vi "Begin.vi"(8 "error in":errorcluster) -> (0 "error out":errorcluster)   [LabVIEW 2017]
doc: "Called before other user functions, this VI is expected to open initial I/O refnums, load in file data, and do all program initialization. Notice that the <B>error out</B> terminal is simply used for data flow. Wiring it to other structures or subVIs ensures that this VI runs first."
uses:
  <vilib>/Rock Robotics/WPI/DriverStation/WPI_DriverStationRobotMode2.ctl
  <vilib>/Rock Robotics/WPI/Joystick/WPI_JoystickDeviceEnum.ctl
  <vilib>/Rock Robotics/WPI/ThirdParty/Phoenix-LabVIEW/Motor Controller/Controls/CTRE_Phoenix_MotorControl_ControlMode.ctl
  <vilib>/Rock Robotics/WPI/ThirdParty/Phoenix-LabVIEW/CANifier/CTRE_CANifier_StatusFrame.ctl
  <vilib>/Rock Robotics/WPI/ThirdParty/Phoenix-LabVIEW/Motor Controller/Controls/CTRE_Phoenix_MotorControl_FeedbackDevice.ctl
  Robot Global Data.vi
  <vilib>/Rock Robotics/WPI/ThirdParty/Phoenix-LabVIEW/Pigeon IMU/CTRE_PigeonIMU_Open_CAN.vi
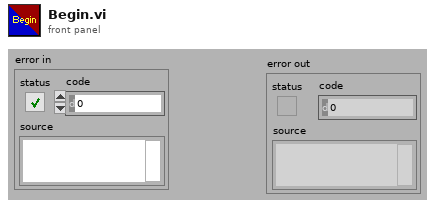
[diagram p1: front panel]
types:
  T1 = typedef "CTRE_Phoenix_MotorControl_FeedbackDevice.ctl" = i8
  T2 = typedef "CTRE_CANifier_StatusFrame.ctl" = u32
  T3 = typedef "CTRE_Phoenix_MotorControl_ControlMode.ctl" = u16
  T4 = typedef "WPI_JoystickDeviceEnum.ctl" = enum16{"USB 0", "USB 1", "USB 2", "USB 3", "USB 4", "USB 5"}
  T5 = typedef "WPI_DriverStationRobotMode2.ctl" = enum16{"Autonomous Disabled", "Autonomous Enabled", "Teleop Disabled", "Teleop Enabled", "Disconnected", "Finish", "Test Disabled", "Test Enabled", "Emergency Stopped"}
  T6 = typedef "WPI_JoystickDevRef.ctl" = cluster{"Device":T4}
  T7 = typedef "CTRE_PigeonIMU_DeviceRef.ctl" = cluster{"DeviceStatus":errorcluster, "Device Number":u8, "Type":T8, "Device ID":u32, "Handle":u64, "UsageFrame":u32, "Library Path":path}
  T8 = typedef "CTRE_PigeonIMU_ConnectionType.ctl" = u32
  T9 = typedef "WPI_MotorControlDeviceRef.ctl" = cluster{"DeviceStatus":errorcluster, "Type":T10, "PWM":cluster{"PWM Channel":T11, "DeadBand":T12}, "CAN":cluster{"Device Number":u8, "SetOutput VI Ref":variant, "GetOutput VI Ref":variant, "Enable VI Ref":variant, "Disable VI Ref":variant, "Data":variant}, "Invert":bool, "DIO PWM":cluster{"PWM \"Enable\" Channel":T11, "DIOChannel":T13, "PWM Rate":dbl}}
  T10 = typedef "WPI_MotorControlType.ctl" = enum16{"PWM", "CAN", "DIO PWM"}
  T11 = typedef "FPGA_DIOPWMChannel.ctl" = enum8{"PWM 0", "PWM 1", "PWM 2", "PWM 3", "PWM 4", "PWM 5", "PWM 6", "PWM 7", "PWM 8", "PWM 9", "PWM MXP 0", "PWM MXP 1", "PWM MXP 2", "PWM MXP 3", "PWM MXP 4", "PWM MXP 5", "PWM MXP 6", "PWM MXP 7", "PWM MXP 8", "PWM MXP 9", "Invalid"}
  T12 = typedef "WPI_PWMDeadband.ctl" = cluster{"Name":string, "maxPositivePwm":i32, "minPositivePwm":i32, "centerPwm":i32, "maxNegativePwm":i32, "minNegativePwm":i32, "angularRange":u16}
  T13 = typedef "FPGA_DIOChannel.ctl" = enum8{"DIO 0", "DIO 1", "DIO 2", "DIO 3", "DIO 4", "DIO 5", "DIO 6", "DIO 7", "DIO 8", "DIO 9", "DIO MXP 0", "DIO MXP 1", "DIO MXP 2", "DIO MXP 3", "DIO MXP 4", "DIO MXP 5", "DIO MXP 6", "DIO MXP 7", "DIO MXP 8", "DIO MXP 9", "DIO MXP 10", "DIO MXP 11", "DIO MXP 12", "DIO MXP 13", "DIO MXP 14", "DIO MXP 15", "SPI Port CS1", "SPI Port CS2", "SPI Port CS3", "SPI Port MISO", "SPI Port MOSI", "Invalid"}
  T14 = typedef "CTRE_CANifier_DeviceRef.ctl" = cluster{"DeviceStatus":errorcluster, "Device Number":u8, "Handle":u64, "UsageFrame":u32, "Library Path":path}
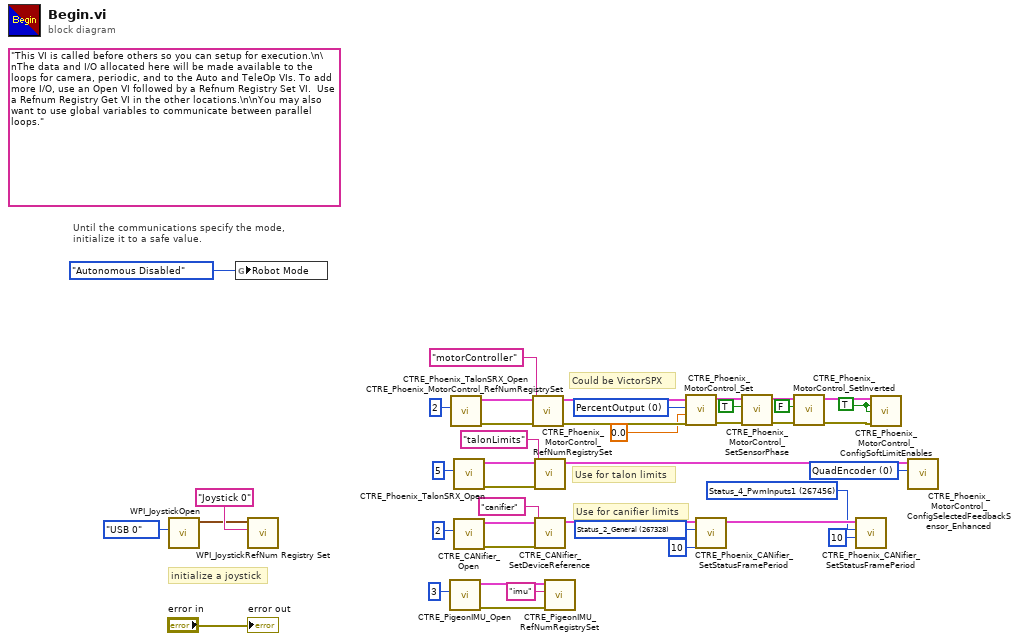
[diagram p0: block diagram]
diagram:
  w4 = T1 0 items=["None"=-1, "QuadEncoder"=0, "Analog"=2, "Tachometer"=4, "Pulse Width Encoded Position"=8, "Sensor Sum (S0 + S1)"=9, "Sensor Difference (D0 - D1)"=10, "Remote Source 0"=11, "Remote Source 1"=12, "Software Emulated"=15] ("Feedback Device")
  w1 = TRUE ("Override Soft Limit Enable?")
  w7 = T2 267456 items=["Status_1_General"=267264, "Status_2_General"=267328, "Status_3_PwmInputs0"=267392, "Status_4_PwmInputs1"=267456, "Status_5_PwmInputs2"=267520, "Status_6_PwmInputs3"=267584, "Status_8_Misc"=267712] ("CANifier Status Frame")
  w10 = T2 267328 items=["Status_1_General"=267264, "Status_2_General"=267328, "Status_3_PwmInputs0"=267392, "Status_4_PwmInputs1"=267456, "Status_5_PwmInputs2"=267520, "Status_6_PwmInputs3"=267584, "Status_8_Misc"=267712] ("CANifier Status Frame")
  w23 = T3 0 items=["PercentOutput"=0, "Position"=1, "Velocity"=2, "Current"=3, "Follower"=5, "MotionProfile"=6, "MotionMagic"=7, "MotionMagicArc"=8, "MotionProfileArc"=10, "Disabled"=15] ("Control Mode")
  (unwired) "This VI is called before others so you can setup for execution.\n\nThe data and I/O allocated here will be made available to the loops for camera, periodic, and to the Auto and TeleOp VIs. To add more I/O, use an Open VI followed by a Refnum Registry Set VI.  Use a Refnum Registry Get VI in the other locations.\n\nYou may also want to use global variables to communicate between parallel loops."
  # "Use for canifier limits"
  # "Use for talon limits"
  # "Could be VictorSPX"
  # "initialize a joystick"
  # "Until the communications specify the mode,\ninitialize it to a safe value."
  n1 = call <vilib>:"WPI_JoystickOpen.vi"("JoystickDevice"=WPI_JoystickDeviceEnum."USB 0") -> ("JoystickDevRef"=w40:T6)  [unwired: 10 in]
  n2 = global write "Robot Global Data.vi" "Robot Mode"(WPI_DriverStationRobotMode2."Autonomous Disabled" ("Robot Mode")) -> ()
  n3 = call <vilib>:"WPI_JoystickRefNum Registry Set.vi"("refnum name"="Joystick 0", "JoystickDevRef"=w40) -> ()  [unwired: 8 in, 2 out]
  n4 = call-poly <vilib>:"CTRE_PigeonIMU_Open.vi"("Device Number"=u8 3) -> ("error out"=w20:errorcluster, "PigeonIMUDevRef"=w19:T7)  [unwired: 9 in]
  n5 = call <vilib>:"CTRE_Phoenix_TalonSRX_Open.vi"("Device Number"=u8 2) -> ("error out"=w36:errorcluster, "CAN Talon SRX Ref"=w35:T9)  [unwired: 9 in]
  n6 = call <vilib>:"CTRE_Phoenix_TalonSRX_Open.vi"("Device Number"=u8 5) -> ("error out"=w32:errorcluster, "CAN Talon SRX Ref"=w31:T9)  [unwired: 9 in]
  n7 = call <vilib>:"CTRE_CANifier_Open.vi"("Device Number"=u8 2) -> ("error out"=w28:errorcluster, "CANifierDevRef"=w27:T14)  [unwired: 9 in]
  n8 = call <vilib>:"CTRE_Phoenix_MotorControl_RefNumRegistrySet.vi"("error in (no error)"=w36, "refnum name"="motorController", "PhoenixMotorControlDevRef"=w35) -> ("error out"=w25:errorcluster, "PhoenixMotorControlDevRef"=w24:T9)  [unwired: 7 in]
  n9 = call <vilib>:"CTRE_Phoenix_MotorControl_RefNumRegistrySet.vi"("error in (no error)"=w32, "refnum name"="talonLimits", "PhoenixMotorControlDevRef"=w31) -> ("PhoenixMotorControlDevRef"=w5:T9)  [unwired: 7 in, 1 out]
  n10 = call <vilib>:"CTRE_CANifier_SetDeviceReference.vi"("error in (no error)"=w28, "refnum name"="canifier", "CANifierDevRef"=w27) -> ("CANifierDevRef"=w11:T14)  [unwired: 7 in, 1 out]
  n11 = call <vilib>:"CTRE_PigeonIMU_RefNumRegistrySet.vi"("error in (no error)"=w20, "refnum name"="imu", "PigeonIMUDevRef"=w19) -> ()  [unwired: 7 in, 2 out]
  n12 = call <vilib>:"CTRE_Phoenix_MotorControl_Set.vi"("error in (no error)"=w25, "Output"=0.0, "Control Mode"=w23, "PhoenixMotorControlDevRef"=w24) -> ("error out"=w17:errorcluster, "PhoenixMotorControlDevRef"=w16:T9)  [unwired: 6 in]
  n13 = call <vilib>:"CTRE_Phoenix_CANifier_SetStatusFramePeriod.vi"("periodMs"=10, "CANifier Status Frame"=w10, "CANifierDevRef"=w11) -> ("CANifierDevRef"=w8:T14)  [unwired: 7 in, 1 out]
  n14 = call <vilib>:"CTRE_Phoenix_MotorControl_SetSensorPhase.vi"("error in (no error)"=w17, "PhaseSensor"=TRUE, "PhoenixMotorControlDevRef"=w16) -> ("error out"=w14:errorcluster, "PhoenixMotorControlDevRef"=w13:T9)  [unwired: 7 in]
  n15 = call <vilib>:"CTRE_Phoenix_MotorControl_SetInverted.vi"("error in (no error)"=w14, "Invert?"=FALSE, "PhoenixMotorControlDevRef"=w13) -> ("error out"=w2:errorcluster, "PhoenixMotorControlDevRef"=w3:T9)  [unwired: 7 in]
  n16 = call <vilib>:"CTRE_Phoenix_CANifier_SetStatusFramePeriod.vi"("periodMs"=10, "CANifier Status Frame"=w7, "CANifierDevRef"=w8) -> ()  [unwired: 7 in, 2 out]
  n17 = call <vilib>:"CTRE_Phoenix_MotorControl_ConfigSoftLimitEnables.vi"("PhoenixMotorControlDevRef"=w3, "Forward Soft Limit Enable"=w1, "Reverse Soft Limit Enable"=w1, "error in (no error)"=w2) -> ()  [unwired: 10 in, 2 out]
  n18 = call <vilib>:"CTRE_Phoenix_MotorControl_ConfigSelectedFeedbackSensor_Enhanced.vi"("Feedback Device"=w4, "PhoenixMotorControlDevRef"=w5) -> ()  [unwired: 8 in, 2 out]
  "error out" <- "error in"
